vi "Save_data.vi"() -> ()   [LabVIEW 2015]
panel:
  in  "Measurement Arrays":T1
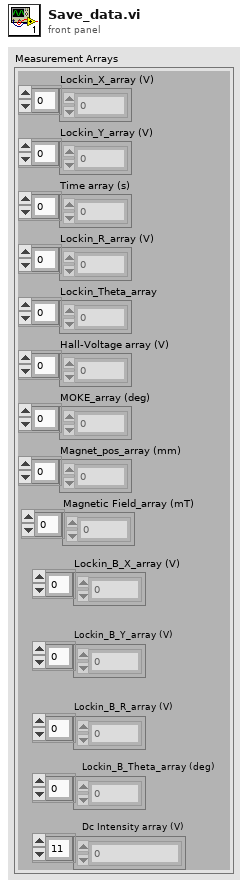
[diagram p1: front panel]
types:
  T1 = cluster{"Lockin_X_array (V)":dbl[], "Lockin_Y_array (V)":dbl[], "Time array (s)":dbl[], "Lockin_R_array (V)":dbl[], "Lockin_Theta_array":dbl[], "Hall-Voltage array (V)":dbl[], "MOKE_array (deg)":dbl[], "Magnet_pos_array (mm)":dbl[], "Magnetic Field_array (mT)":dbl[], "Lockin_B_X_array (V)":dbl[], "Lockin_B_Y_array (V)":dbl[], "Lockin_B_R_array (V)":dbl[], "Lockin_B_Theta_array (deg)":dbl[], "Dc Intensity array (V)":dbl[]}
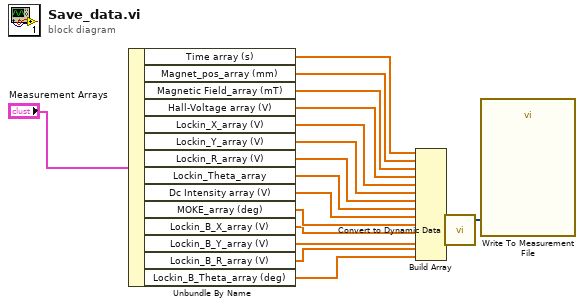
[diagram p0: block diagram]
diagram:
  n1 = Unbundle By Name("Measurement Arrays") -> ("Time array (s)"=w11:dbl[], "Magnet_pos_array (mm)"=w15:dbl[], "Magnetic Field_array (mT)"=w14:dbl[], "Hall-Voltage array (V)"=w13:dbl[], "Lockin_X_array (V)"=w10:dbl[], "Lockin_Y_array (V)"=w9:dbl[], "Lockin_R_array (V)"=w8:dbl[], "Lockin_Theta_array"=w7:dbl[], "Dc Intensity array (V)"=w6:dbl[], "MOKE_array (deg)"=w5:dbl[], "Lockin_B_X_array (V)"=w4:dbl[], "Lockin_B_Y_array (V)"=w3:dbl[], "Lockin_B_R_array (V)"=w2:dbl[], "Lockin_B_Theta_array (deg)"=w1:dbl[])
  n2 = Build Array(w11, w15, w14, w13, w10, w9, w8, w7, w6, w5, w4, w3, w2, w1) -> (w17:dbl[][])
  n3 = call "Convert to Dynamic Data"("2D Array"=w17) -> ("Dynamic Data Type"=w16:dynamicdata)  [unwired: 3 in]
  n4 = call "Write To Measurement File"("Signals"=w16) -> ()  [unwired: 16 in, 3 out]
